vi "NET_SRX_Amperage.vi"(8 "Read(F) Write(T)":bool, 11 "SRX_Amp_Cluster":T1) -> (3 "SRX_Amp_Cluster Out":T1)   [LabVIEW 2017]
uses:
  TypeDef/Cluster_SRX_Amperage.ctl
  <vilib>/Rock Robotics/Network Tables/NT Read Numeric Array.vi
  <vilib>/Rock Robotics/Network Tables/NT Write Numeric Array.vi
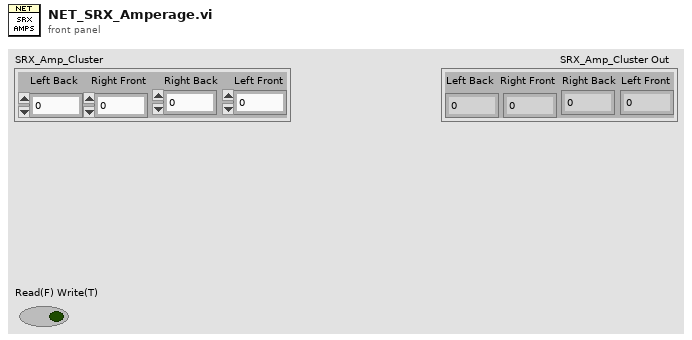
[diagram p1: front panel]
types:
  T1 = typedef "Cluster_SRX_Amperage.ctl" = cluster{"Left Back":dbl, "Right Front":dbl, "Right Back":dbl, "Left Front":dbl}
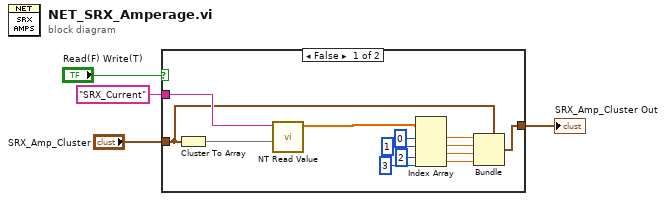
[diagram p0: block diagram]
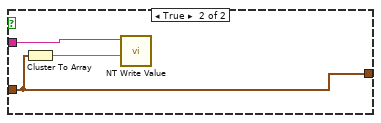
[diagram p2: hidden frame]
diagram:
  n1 = case shown="False" "Read(F) Write(T)" {
    tunnel: "SRX_Amp_Cluster" -> [w10 w18]
    tunnel: "SRX_Current" ("Name") -> [w17 w19]
    tunnel: [w5 w18] -> w1
    frame False {
      n2 = Cluster To Array(cluster=w10) -> (array=w16:dbl[])
      n3 = call-poly <vilib>:"NT Read Value.vi"("Default Value"=w16, "Name"=w17) -> ("Numeric Array"=w15:dbl[])  [unwired: 8 in, 1 out]
      n4 = Index Array(array=w15, index #1=0 ("index"), index #2=1 ("index"), index #3=2 ("index"), index #4=3 ("index")) -> (element #1=w14:dbl, element #2=w13:dbl, element #3=w12:dbl, element #4=w11:dbl)
      n5 = Bundle(cluster=w10, "Left Back"=w14, "Right Front"=w13, "Right Back"=w12, "Left Front"=w11) -> (w5:T1)
    }
    frame True {
      n6 = Cluster To Array(cluster=w18) -> (array=w20:dbl[])
      n7 = call-poly <vilib>:"NT Write Value.vi"("Numeric Array"=w20, "Name"=w19) -> ()  [unwired: 9 in, 1 out]
    }
  }
  "SRX_Amp_Cluster Out" <- w1
